vi "Create Waveform Cluster.vi"(8 "error in":errorcluster, 11 "Node":refnum<k20>) -> (0 "error out":errorcluster, 1 "Clust Refnum":refnum<vi>, 2 "Waveform Type":string, 3 "Node":refnum<k20>)   [LabVIEW 2026, in "Plugin XML Parser.lvlib"]
uses:
  Plugin XML Parser.lvlib
  <vilib>/numeric/LVNumericRepresentation.ctl
  <vilib>/Utility/miscctls.llb/LVPositionTypeDef.ctl
  <vilib>/xml/Close Reference(Node).vi
  <resource>/objmgr/DOMUserDefRef.rc
  <vilib>/xml/NI_XML.lvlib
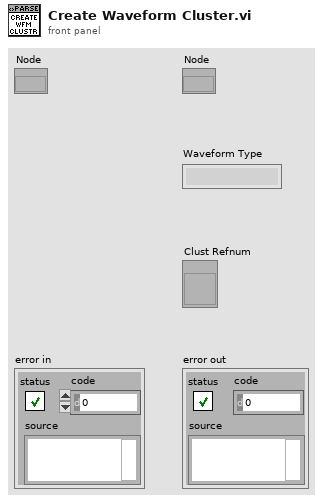
[diagram p1: front panel]
types:
  T1 = typedef "LVNumericRepresentation.ctl" = enum32{"Extended Precision", "Double Precision", "Single Precision", "Long", "Word", "Byte", "Unsigned Long", "Unsigned Word", "Unsigned Byte", "Complex Extended", "Complex Double", "Complex Single", "Quad", "Unsigned Quad", "Fixed-Point"}
  T2 = typedef "LVPositionTypeDef.ctl" = cluster{"Left":i32, "Top":i32}
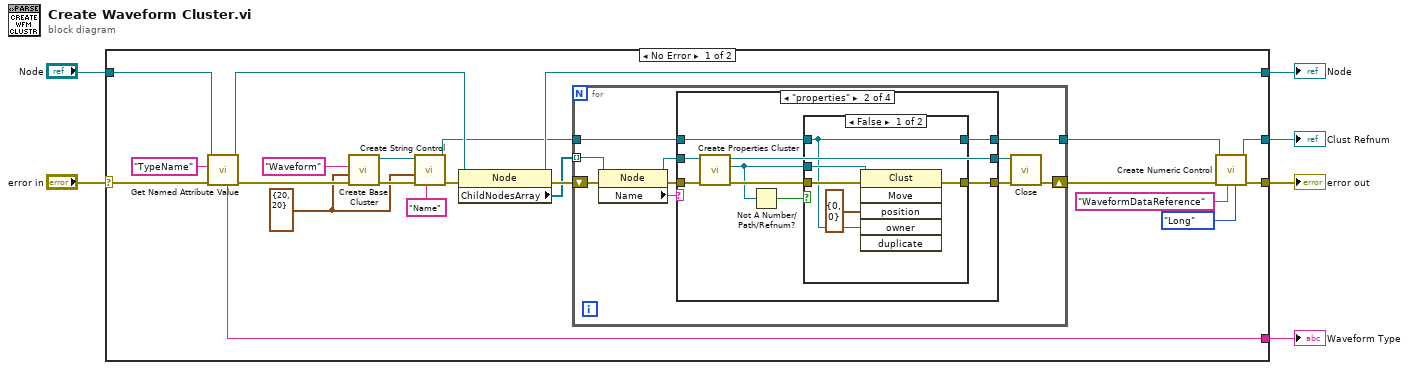
[diagram p0: block diagram]
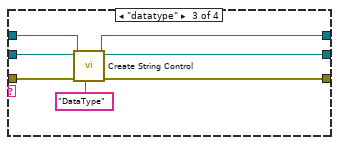
[diagram p4: hidden frame]
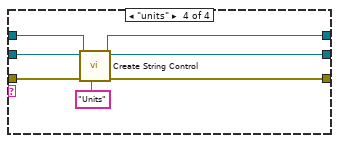
[diagram p5: hidden frame]
diagram:
  n1 = case shown="No Error" "error in" {
    selector: "error in" -> [w23 w71]
    tunnel: [w7 w71] -> w6
    tunnel: [w27 w70] -> w4
    tunnel: "Node" -> [w25 w70]
    tunnel: [w10 _] -> w2
    tunnel: [w22 _] -> w1
    frame No Error {
      w14 = cluster{"Horizontal":i16, "Vertical":i16} {"Horizontal"=20, "Vertical"=20} ("Point")
      n2 = call "Get Named Attribute Value.vi"("error in"=w23, "Attribute Name"="TypeName", "Node In"=w25) -> ("error out"=w20:errorcluster, "Node Out"=w24:refnum<k20>, "Attribute Value"=w22:string)  [unwired: 5 in, 1 out]
      n3 = call "Create Base Cluster.vi"("error in"=w20, "Location"=w14, "Cluster Name"="Waveform") -> ("error out"=w16:errorcluster, "Cluster out"=w18:refnum<vi>)  [unwired: 6 in, 1 out]
      n4 = call "Create String Control.vi"("Label.Text"="Name", "error in"=w16, "location"=w14, "Cluster in"=w18) -> ("error out"=w15:errorcluster, "Cluster out"=w17:refnum<vi>)  [unwired: 6 in]
      n5 = property class="Node"(reference=w24, error in=w15) -> (reference out=w27:refnum<k20>, error out=w28:errorcluster, "ChildNodesArray"=w26:refnum<k20>[])
      n6 = for {
        tunnel: w26 -> [w34] mode=indexing
        shift-right: [w35] -> w12
        shift-left: w28 -> [w38]
        tunnel: w17 -> [w30]
        tunnel: [w29] -> w11
        n7 = property class="Node"(reference=w34, error in=w38) -> (reference out=w32:refnum<k20>, error out=w37:errorcluster, "Name"=w33:string)
        n8 = case shown="\"properties\"" w33 {
          tunnel: w32 -> [w40 w47 w58 w64]
          tunnel: [w40 w46 w58 w64] -> w31
          tunnel: w37 -> [w41 w50 w63 w69]
          tunnel: w30 -> [w39 w44 w61 w67]
          tunnel: [w41 w48 w62 w68] -> w36
          tunnel: [w39 w42 w60 w66] -> w29
          frame Default {
          }
          frame "properties" {
            n9 = call "Create Properties Cluster.vi"("error in"=w50, "Node In"=w47) -> ("error out"=w49:errorcluster, "Clust Refnum"=w45:refnum<vi>, "Node Out"=w46:refnum<k20>)  [unwired: 7 in]
            n10 = Not A Number/Path/Refnum?(number/path/refnum=w45) -> (NaN/Path/Refnum?=w43:bool)
            n11 = case shown="False" w43 {
              tunnel: w44 -> [w51 w56]
              tunnel: w49 -> [w55 w57]
              tunnel: [w54 w57] -> w48
              tunnel: w45 -> [w52 _]
              tunnel: [w51 w56] -> w42
              frame False {
                n12 = invoke class="Clust" method="Move"(reference=w52, error in=w55, "position"=T2 {"Left"=0, "Top"=0}, "owner"=w51) -> (error out=w54:errorcluster)  [unwired: 2 in, 5 out]
              }
              frame True {
              }
            }
          }
          frame "datatype" {
            n13 = call "Create String Control.vi"("Label.Text"="DataType", "error in"=w63, "Cluster in"=w61) -> ("error out"=w62:errorcluster, "Cluster out"=w60:refnum<vi>)  [unwired: 7 in]
          }
          frame "units" {
            n14 = call "Create String Control.vi"("Label.Text"="Units", "error in"=w69, "Cluster in"=w67) -> ("error out"=w68:errorcluster, "Cluster out"=w66:refnum<vi>)  [unwired: 7 in]
          }
        }
        n15 = call-poly <vilib>:"Close.vi"("error in (no error)"=w36, "node"=w31) -> ("error out"=w35:errorcluster)  [unwired: 7 in]
      }
      n16 = call "Create Numeric Control.vi"("Representation"=LVNumericRepresentation."Long", "Label.Text"="WaveformDataReference", "error in"=w12, "Cluster in"=w11) -> ("error out"=w7:errorcluster, "Cluster out"=w10:refnum<vi>)  [unwired: 6 in]
    }
    frame Error {
    }
  }
  "Node" <- w4
  "error out" <- w6
  "Waveform Type" <- w1
  "Clust Refnum" <- w2
